vi "Example1.vi"() -> ()   [LabVIEW 2019]
uses:
  VGrid_class/VGrid.lvclass
  C:/Users/Taylor.Hillegeist/OneDrive - Ultra/LabVIEW/Pgui2/Pgui_Obj_class/Pgui_Obj.lvclass
  Button_class/Button.lvclass
  SparkLine_class/SparkLine.lvclass
  HGrid_class/HGrid.lvclass
  Digital_class/Digital.lvclass
panel:
  out "Rectangles":string
  out "2D Picture":picture
  out "Click Event":string
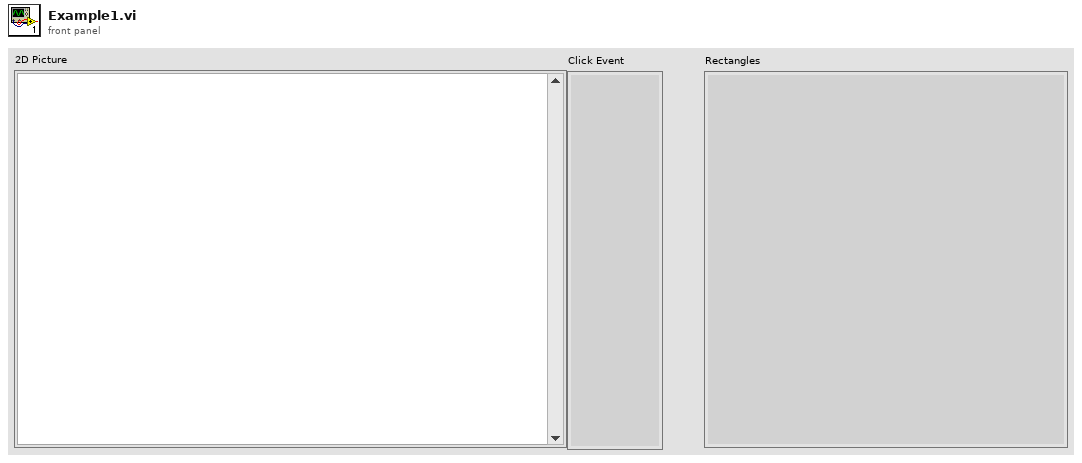
[diagram p1: front panel]
types:
  T1 = typedef "LVMouseTypeDef.ctl" = cluster{"Mouse Position":cluster{"X":i32, "Y":i32}, "Mouse Modifiers":cluster{"Button Down":bool, "Shift Mod":bool, "Menu Mod":bool, "Option Mod":bool}}
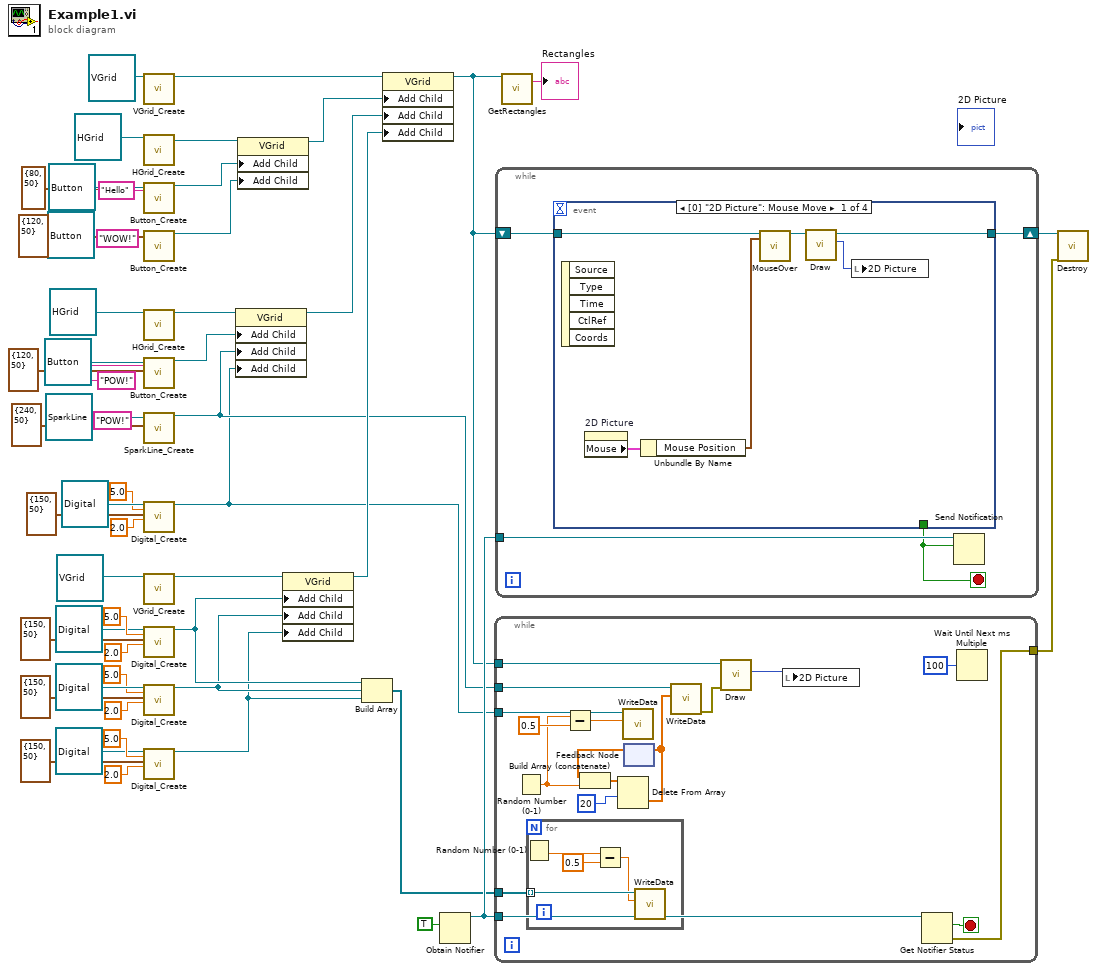
[diagram p0: block diagram]
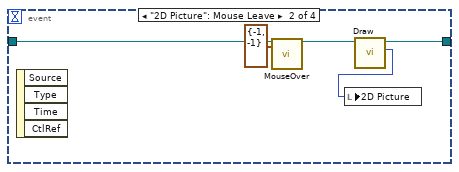
[diagram p2: hidden frame]
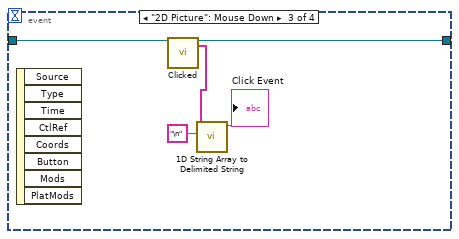
[diagram p3: hidden frame]
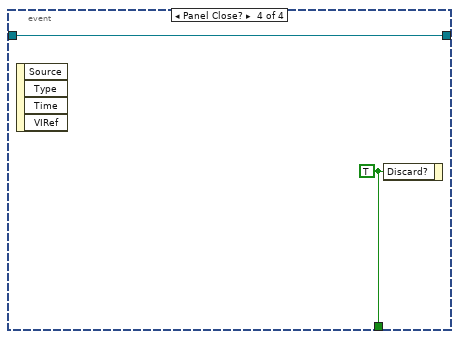
[diagram p4: hidden frame]
diagram:
  (unwired) "POW!" ("Text")
  n1 = call "VGrid_Create.vi"("reference in"=refnum<class "VGrid.lvclass"> refnum ("VGrid")) -> ("reference out"=w7:refnum<class "VGrid.lvclass">)  [unwired: 17 in, 1 out]
  n2 = call "HGrid_Create.vi"("reference in"=refnum<class "HGrid.lvclass"> refnum ("VGrid")) -> ("reference out"=w26:refnum<class "HGrid.lvclass">)  [unwired: 17 in, 1 out]
  n3 = call "Button_Create.vi"("reference in"=refnum<class "Button.lvclass"> refnum, "Text"="Hello", "Override size"=cluster{"Width":i16, "Height":i16} {"Width"=80, "Height"=50}) -> ("reference out"=w25:refnum<class "Button.lvclass">)  [unwired: 15 in, 1 out]
  n4 = call "Button_Create.vi"("reference in"=refnum<class "Button.lvclass"> refnum, "Text"="WOW!", "Override size"=cluster{"Width":i16, "Height":i16} {"Width"=120, "Height"=50}) -> ("reference out"=w24:refnum<class "Button.lvclass">)  [unwired: 15 in, 1 out]
  n5 = call "HGrid_Create.vi"("reference in"=refnum<class "HGrid.lvclass"> refnum ("VGrid")) -> ("reference out"=w23:refnum<class "HGrid.lvclass">)  [unwired: 17 in, 1 out]
  n6 = call "Button_Create.vi"("reference in"=refnum<class "Button.lvclass"> refnum, "Text"="POW!", "Override size"=cluster{"Width":i16, "Height":i16} {"Width"=120, "Height"=50}) -> ("reference out"=w22:refnum<class "Button.lvclass">)  [unwired: 15 in, 1 out]
  n7 = call "SparkLine_Create.vi"("reference in"=refnum<class "SparkLine.lvclass"> refnum, "Override size"=cluster{"Width":i16, "Height":i16} {"Width"=240, "Height"=50}) -> ("reference out"=w2:refnum<class "SparkLine.lvclass">)  [unwired: 16 in, 1 out]
  n8 = call "Digital_Create.vi"("reference in"=refnum<class "Digital.lvclass"> refnum ("Pgui_Button"), "Digits Total"=5.0, "Override size"=cluster{"Width":i16, "Height":i16} {"Width"=150, "Height"=50}, "Digits Precision"=2.0) -> ("reference out"=w1:refnum<class "Digital.lvclass">)  [unwired: 14 in, 1 out]
  n9 = call "VGrid_Create.vi"("reference in"=refnum<class "VGrid.lvclass"> refnum ("VGrid")) -> ("reference out"=w29:refnum<class "VGrid.lvclass">)  [unwired: 17 in, 1 out]
  n10 = call "Digital_Create.vi"("reference in"=refnum<class "Digital.lvclass"> refnum ("Pgui_Button"), "Digits Total"=5.0, "Override size"=cluster{"Width":i16, "Height":i16} {"Width"=150, "Height"=50}, "Digits Precision"=2.0) -> ("reference out"=w28:refnum<class "Digital.lvclass">)  [unwired: 14 in, 1 out]
  n11 = call "Digital_Create.vi"("reference in"=refnum<class "Digital.lvclass"> refnum ("Pgui_Button"), "Digits Total"=5.0, "Override size"=cluster{"Width":i16, "Height":i16} {"Width"=150, "Height"=50}, "Digits Precision"=2.0) -> ("reference out"=w13:refnum<class "Digital.lvclass">)  [unwired: 14 in, 1 out]
  n12 = call "Digital_Create.vi"("reference in"=refnum<class "Digital.lvclass"> refnum ("Pgui_Button"), "Digits Total"=5.0, "Override size"=cluster{"Width":i16, "Height":i16} {"Width"=150, "Height"=50}, "Digits Precision"=2.0) -> ("reference out"=w12:refnum<class "Digital.lvclass">)  [unwired: 14 in, 1 out]
  n13 = property class="VGrid"(reference=w23, "Add Child"=w22, "Add Child"=w2, "Add Child"=w1) -> (reference out=w4:refnum<class "HGrid.lvclass">)  [unwired: 1 in, 1 out]
  n14 = property class="VGrid"(reference=w26, "Add Child"=w25, "Add Child"=w24) -> (reference out=w5:refnum<class "HGrid.lvclass">)  [unwired: 1 in, 1 out]
  n15 = property class="VGrid"(reference=w29, "Add Child"=w28, "Add Child"=w13, "Add Child"=w12) -> (reference out=w3:refnum<class "VGrid.lvclass">)  [unwired: 1 in, 1 out]
  n16 = Build Array(w28, w13, w12) -> (w27:refnum<class "Digital.lvclass">[])
  n17 = property class="VGrid"(reference=w7, "Add Child"=w5, "Add Child"=w4, "Add Child"=w3) -> (reference out=w6:refnum<class "VGrid.lvclass">)  [unwired: 1 in, 1 out]
  n18 = Obtain Notifier(notification data type=TRUE) -> (notifier out=w40:refnum<notifier>)  [unwired: 3 in, 2 out]
  n19 = while {
    tunnel: w2 -> [w70]
    tunnel: w40 -> [w68]
    tunnel: w6 -> [w66]
    tunnel: [w65] -> w36
    tunnel: w1 -> [w64]
    tunnel: w27 -> [w61]
    stop <- w69 stop-if-true
    n20 = Random Number (0-1)() -> (number: 0 to 1=w56:dbl)
    n21 = for {
      tunnel: w61 -> [w74] mode=indexing
      n22 = Random Number (0-1)() -> (number: 0 to 1=w72:dbl)
      n23 = Subtract(x=w72, y=0.5) -> (x-y=w71:dbl)
      n24 = call-dynamic "WriteData.vi"("Value"=w71, "reference in"=w74) -> ()  [unwired: 8 in, 2 out]
    }
    n25 = Subtract(x=w56, y=0.5) -> (x-y=w63:dbl)
    n26 = call-dynamic "WriteData.vi"("Value"=w63, "reference in"=w64) -> ()  [unwired: 8 in, 2 out]
    n27 = feedback #1() -> (w58:dbl[])  [unwired: 1 in]
    n28 = Build Array (concatenate)(w58, w56) -> (w57:dbl[])
    n29 = Delete From Array(array=w57, length=20) -> (deleted portion=w55:dbl[])  [unwired: 1 in, 1 out]
    n30 = feedback-in #1(w55) -> ()
    n31 = call-dynamic "WriteData.vi"("Data"=w55, "reference in"=w70) -> ("error out"=w62:errorcluster)  [unwired: 8 in, 1 out]
    n32 = call-dynamic "Draw.vi"("error in (no error)"=w62, "reference in"=w66) -> ("Draw Instr"=w67:picture)  [unwired: 7 in, 2 out]
    n33 = local write "2D Picture"(w67) -> ()
    n34 = Get Notifier Status(notifier=w68) -> (current notification=w69:bool, error out=w65:errorcluster)  [unwired: 1 in, 3 out]
    n35 = Wait Until Next ms Multiple(millisecond multiple=u32 100) -> ()  [unwired: 1 out]
  }
  n36 = while {
    shift-right: [w77] -> w52
    shift-left: w6 -> [w78]
    tunnel: w40 -> [w76]
    stop <- w75 stop-if-true
    n37 = event shown="[0] \"2D Picture\": Mouse Move" {
      selector: _ -> [_ _ _ _]
      dyn-events: _ -> [_ _ _ _]
      timeout: _ -> [_ _ _ _]
      tunnel: w78 -> [w84 w89 w94 w95]
      tunnel: [w82 w87 w90 w95] -> w77
      tunnel: [_ _ _ w96] -> w75
      event "2D Picture": Mouse Move {
        n38 = event-data() -> ()  [unwired: 1 in, 5 out]
        n39 = property on="2D Picture" class="Pict"() -> ("Mouse"=w79:T1)  [unwired: 2 in, 2 out]
        n40 = Unbundle By Name(w79) -> ("Mouse Position"=w80:cluster{"X":i32, "Y":i32})
        n41 = call-dynamic "MouseOver.vi"("reference in"=w84, "point"=w80) -> ("reference out"=w83:refnum<class "VGrid.lvclass">)  [unwired: 16 in, 1 out]
        n42 = call-dynamic "Draw.vi"("reference in"=w83) -> ("Draw Instr"=w81:picture, "reference out"=w82:refnum<class "VGrid.lvclass">)  [unwired: 8 in, 1 out]
        n43 = local write "2D Picture"(w81) -> ()
      }
      event "2D Picture": Mouse Leave {
        n44 = event-data() -> ()  [unwired: 1 in, 4 out]
        n45 = call-dynamic "MouseOver.vi"("reference in"=w89, "point"=cluster{"x":i16, "y":i16} {"x"=-1, "y"=-1}) -> ("reference out"=w88:refnum<class "VGrid.lvclass">)  [unwired: 16 in, 1 out]
        n46 = call-dynamic "Draw.vi"("reference in"=w88) -> ("Draw Instr"=w86:picture, "reference out"=w87:refnum<class "VGrid.lvclass">)  [unwired: 8 in, 1 out]
        n47 = local write "2D Picture"(w86) -> ()
      }
      event "2D Picture": Mouse Down {
        n48 = event-data() -> ()  [unwired: 1 in, 8 out]
        n49 = call-dynamic "Clicked.vi"("reference in"=w94) -> ("reference out"=w90:refnum<class "VGrid.lvclass">, "Array"=w93:string[])  [unwired: 16 in, 1 out]
        n50 = call <vilib>:"1D String Array to Delimited String.vi"("delimiter"="\n", "string array"=w93) -> ("delimited string"=→"Click Event":string)  [unwired: 9 in]
      }
      event Panel Close? {
        w96 = TRUE ("Discard?")
        n51 = event-data() -> ()  [unwired: 1 in, 4 out]
        n52 = event-data("Discard?"=w96) -> ()  [unwired: 1 in, 1 out]
      }
    }
    n53 = Send Notification(notification=w75, notifier=w76) -> ()  [unwired: 1 in, 2 out]
  }
  n54 = call-dynamic "GetRectangles.vi"("reference in"=w6) -> ("Rectangles"=→"Rectangles":string)  [unwired: 16 in, 2 out]
  n55 = call-dynamic "Destroy.vi"("reference in"=w52, "error in (no error)"=w36) -> ()  [unwired: 16 in, 2 out]
